vi "Convert Folder of VIs to Image.vi"(8 "error in (no error)":errorcluster, 11 "Folder Path":path) -> (0 "error out":errorcluster)   [LabVIEW 2015]
uses:
  <vilib>/Utility/miscctls.llb/LVPointTypeDef.ctl
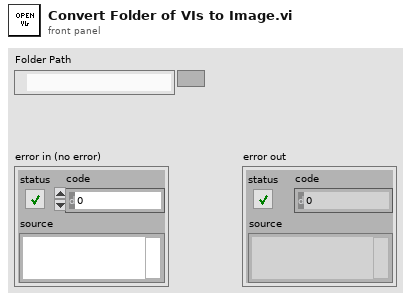
[diagram p1: front panel]
types:
  T1 = typedef "LVPointTypeDef.ctl" = cluster{"Horizontal":i16, "Vertical":i16}
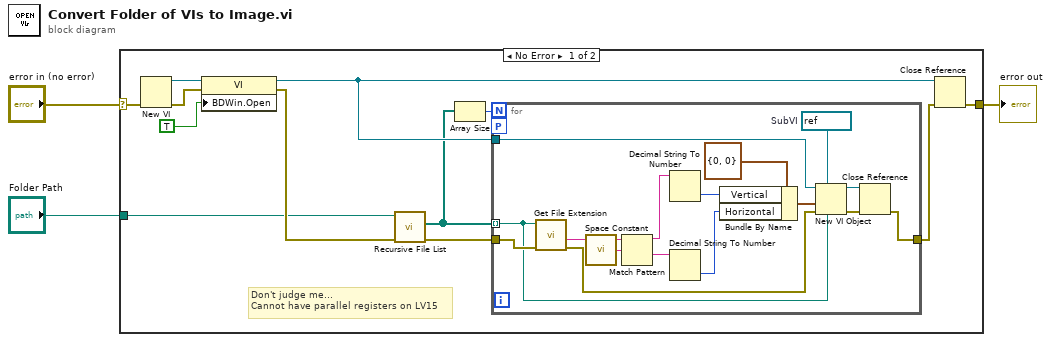
[diagram p0: block diagram]
diagram:
  n1 = case shown="No Error" "error in (no error)" {
    selector: "error in (no error)" -> [w14 w32]
    tunnel: [w11 w32] -> w2
    tunnel: "Folder Path" -> [w8 _]
    frame No Error {
      # "Don't judge me...\nCannot have parallel registers on LV15"
      n2 = New VI(8:w14) -> (0:w13:errorcluster, 3:w7:refnum<vi>)  [unwired: 6 in]
      n3 = property class="VI"(reference=w7, error in=w13, "BDWin.Open"=TRUE ("Block Diagram Window:Open")) -> (reference out=w9:refnum<vi>, error out=w10:errorcluster)
      n4 = call <vilib>:"Recursive File List.vi"("error in (no error)"=w10, "Folder Path"=w8) -> ("error out"=w15:errorcluster, "All Files in Dir"=w4:path[])  [unwired: 5 in, 3 out]
      n5 = Array Size(array=w4) -> (size(s)=w5:i32)
      n6 = for {
        N: w5 -> [_]
        tunnel: w4 -> [w18] mode=indexing
        workers-P: _ -> [_]
        tunnel: w9 -> [w16]
        tunnel: w15 -> [w29]
        tunnel: [w30] -> w12
        w20 = refnum<vi> refnum  # SubVI
        n7 = call <vilib>:"Get File Extension.vi"("error in (no error)"=w29, "file"=w18) -> ("error out"=w28:errorcluster, "filename without extension"=w23:string)  [unwired: 5 in, 3 out]
        n8 = call <vilib>:"Space Constant.vi"() -> ("String"=w22:string)
        n9 = Match Pattern(string=w23, regular expression=w22) -> (before substring=w24:string, after substring=w21:string)  [unwired: 1 in, 2 out]
        n10 = Decimal String To Number(string=w24) -> (number=w25:i32)  [unwired: 2 in, 1 out]
        n11 = Decimal String To Number(string=w21) -> (number=w19:i32)  [unwired: 2 in, 1 out]
        n12 = Bundle By Name(cluster=T1 {"Horizontal"=0, "Vertical"=0} ("location"), "Vertical"=w25, "Horizontal"=w19) -> (w27:T1)
        n13 = New VI Object(vi object class=w20, owner refnum=w16, position/next to=w27, 6:w18, 8:w28) -> (object refnum=w17:refnum<vi>, 0:w31:errorcluster)  [unwired: 3 in]
        n14 = Close Reference(reference=w17, error in (no error)=w31) -> (error out=w30:errorcluster)
      }
      n15 = Close Reference(reference=w9, error in (no error)=w12) -> (error out=w11:errorcluster)
    }
    frame Error {
    }
  }
  "error out" <- w2
